vi "Close File.vi"(8 "error in":errorcluster, 11 "XLS in":refnum<class "XLS.lvclass">) -> (0 "error out":errorcluster, 3 "XLS out":refnum<class "XLS.lvclass">)   [LabVIEW 2017, in "Report_lib.lvlib" / "XLS.lvclass"]
doc: "This Method save & close XLS report"
uses:
  XLS.lvclass
  XLS.lvclass/XLS.ctl
  <vilib>/Utility/NIReport.llb/NI_report.lvclass
  <vilib>/Utility/NIReport.llb/Excel/NI_Excel.lvclass
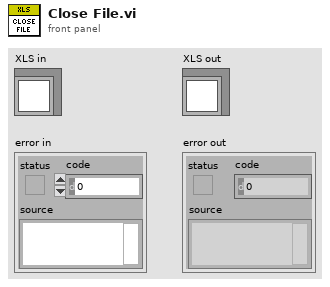
[diagram p1: front panel]
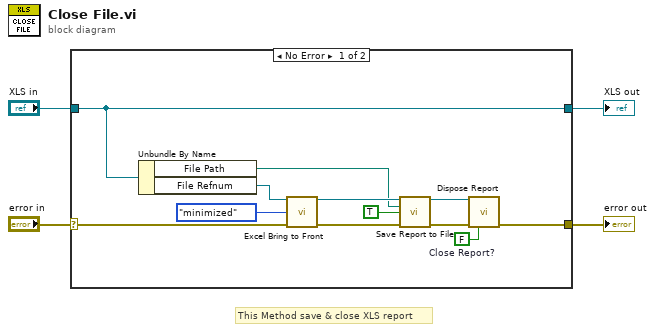
[diagram p0: block diagram]
diagram:
  # "This Method save & close XLS report"
  n1 = case shown="No Error" "error in" {
    selector: "error in" -> [w9 w18]
    tunnel: [w5 w18] -> w3
    tunnel: [w11 w17] -> w1
    tunnel: "XLS in" -> [w11 w17]
    frame No Error {
      w15 = FALSE  # Close Report?
      n2 = Unbundle By Name(w11) -> ("File Path"=w6:path, "File Refnum"=w10:refnum<class "NI_report.lvclass">)
      n3 = call <vilib>:"Excel Bring to Front.vi"("report in"=w10, "window state (maximized)"=enum16{"maximized", "minimized", "normal"}."minimized", "error in (no error)"=w9) -> ("report out"=w7:refnum<class "NI_report.lvclass">, "error out"=w8:errorcluster)  [unwired: 11 in]
      n4 = call-dynamic "Save Report to File.vi"("report in"=w7, "report file path"=w6, "prompt to replace? (F)"=TRUE, "error in (no error)"=w8) -> ("report out"=w13:refnum<class "NI_report.lvclass">, "error out"=w14:errorcluster)  [unwired: 10 in]
      n5 = call-dynamic "Dispose Report.vi"("report in"=w13, "error in (no error)"=w14, "close report? (T)"=w15) -> ("error out"=w5:errorcluster)  [unwired: 12 in]
    }
    frame Error {
    }
  }
  "error out" <- w3
  "XLS out" <- w1
